vi "SubVI_RealAutoDrive_Auto.vi"() -> ()   [LabVIEW 2017]
uses:
  <vilib>/Rock Robotics/WPI/ThirdParty/Phoenix-LabVIEW/Motor Controller/Controls/CTRE_Phoenix_MotorControl_ControlMode.ctl
  <vilib>/Rock Robotics/WPI/ThirdParty/Phoenix-LabVIEW/Motor Controller/Get/CTRE_Phoenix_MotorController_GetSelectedSensorData.vi
panel:
  out "Position(Inches)":dbl
  in  "Output":dbl=1.0
  in  "y":dbl=18.85 format="%#_13g"
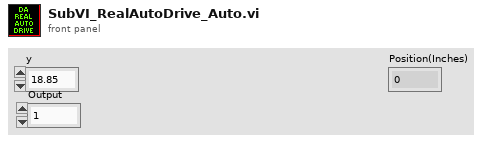
[diagram p1: front panel]
types:
  T1 = typedef "WPI_MotorControlDeviceRef.ctl" = cluster{"DeviceStatus":errorcluster, "Type":T2, "PWM":cluster{"PWM Channel":T3, "DeadBand":T4}, "CAN":cluster{"Device Number":u8, "SetOutput VI Ref":variant, "GetOutput VI Ref":variant, "Enable VI Ref":variant, "Disable VI Ref":variant, "Data":variant}, "Invert":bool, "DIO PWM":cluster{"PWM \"Enable\" Channel":T3, "DIOChannel":T5, "PWM Rate":dbl}}
  T2 = typedef "WPI_MotorControlType.ctl" = enum16{"PWM", "CAN", "DIO PWM"}
  T3 = typedef "FPGA_DIOPWMChannel.ctl" = enum8{"PWM 0", "PWM 1", "PWM 2", "PWM 3", "PWM 4", "PWM 5", "PWM 6", "PWM 7", "PWM 8", "PWM 9", "PWM MXP 0", "PWM MXP 1", "PWM MXP 2", "PWM MXP 3", "PWM MXP 4", "PWM MXP 5", "PWM MXP 6", "PWM MXP 7", "PWM MXP 8", "PWM MXP 9", "Invalid"}
  T4 = typedef "WPI_PWMDeadband.ctl" = cluster{"Name":string, "maxPositivePwm":i32, "minPositivePwm":i32, "centerPwm":i32, "maxNegativePwm":i32, "minNegativePwm":i32, "angularRange":u16}
  T5 = typedef "FPGA_DIOChannel.ctl" = enum8{"DIO 0", "DIO 1", "DIO 2", "DIO 3", "DIO 4", "DIO 5", "DIO 6", "DIO 7", "DIO 8", "DIO 9", "DIO MXP 0", "DIO MXP 1", "DIO MXP 2", "DIO MXP 3", "DIO MXP 4", "DIO MXP 5", "DIO MXP 6", "DIO MXP 7", "DIO MXP 8", "DIO MXP 9", "DIO MXP 10", "DIO MXP 11", "DIO MXP 12", "DIO MXP 13", "DIO MXP 14", "DIO MXP 15", "SPI Port CS1", "SPI Port CS2", "SPI Port CS3", "SPI Port MISO", "SPI Port MOSI", "Invalid"}
  T6 = typedef "CTRE_Phoenix_MotorControl_ControlMode.ctl" = u16
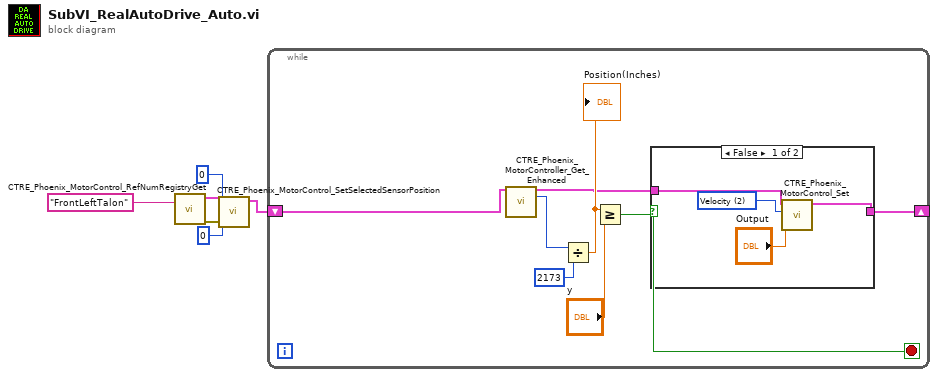
[diagram p0: block diagram]
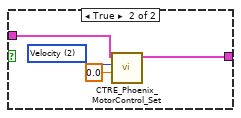
[diagram p2: hidden frame]
diagram:
  n1 = call <vilib>:"CTRE_Phoenix_MotorControl_RefNumRegistryGet.vi"("refnum name"="FrontLeftTalon") -> ("error out"=w3:errorcluster, "PhoenixMotorControlDevRef"=w5:T1)  [unwired: 9 in]
  n2 = call <vilib>:"CTRE_Phoenix_MotorControl_SetSelectedSensorPosition.vi"("error in (no error)"=w3, "pidLoopIdx"=u32 0, "New Sensor Position"=0, "PhoenixMotorControlDevRef"=w5) -> ("PhoenixMotorControlDevRef"=w4:T1)  [unwired: 6 in, 1 out]
  n3 = while {
    shift-right: [w7] -> _
    shift-left: w4 -> [w14]
    stop <- w9 stop-if-true
    n4 = call-poly <vilib>:"CTRE_Phoenix_MotorController_Get_Enhanced.vi"("PhoenixMotorControlDevRef"=w14) -> ("PhoenixMotorControlDevRef"=w8:T1, "Position (Raw Sensor Units)"=w13:i32)  [unwired: 11 in, 2 out]
    n5 = Divide(x=w13, y=2173) -> (x/y=w11:dbl)
    "Position(Inches)" <- w11
    n6 = Greater Or Equal?(x=w11, y="y") -> (x >= y?=w9:bool)
    n7 = case shown="False" w9 {
      tunnel: w8 -> [w17 w22]
      tunnel: [w15 w19] -> w7
      frame False {
        w18 = T6 2 items=["PercentOutput"=0, "Position"=1, "Velocity"=2, "Current"=3, "Follower"=5, "MotionProfile"=6, "MotionMagic"=7, "MotionMagicArc"=8, "MotionProfileArc"=10, "Disabled"=15] ("Control Mode")
        n8 = call <vilib>:"CTRE_Phoenix_MotorControl_Set.vi"("Output"="Output", "Control Mode"=w18, "PhoenixMotorControlDevRef"=w17) -> ("PhoenixMotorControlDevRef"=w15:T1)  [unwired: 7 in, 1 out]
      }
      frame True {
        w20 = T6 2 items=["PercentOutput"=0, "Position"=1, "Velocity"=2, "Current"=3, "Follower"=5, "MotionProfile"=6, "MotionMagic"=7, "MotionMagicArc"=8, "MotionProfileArc"=10, "Disabled"=15] ("Control Mode")
        n9 = call <vilib>:"CTRE_Phoenix_MotorControl_Set.vi"("Output"=0.0, "Control Mode"=w20, "PhoenixMotorControlDevRef"=w22) -> ("PhoenixMotorControlDevRef"=w19:T1)  [unwired: 7 in, 1 out]
      }
    }
  }
